vi "Ex3_Enums.vi"() -> ()   [LabVIEW 2024]
panel:
  in  "OK Button 2":bool
  out "Numeric 3":dbl
  in  "Numeric 2":dbl
  in  "Numeric":dbl
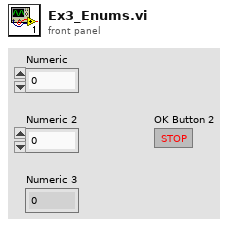
[diagram p1: front panel]
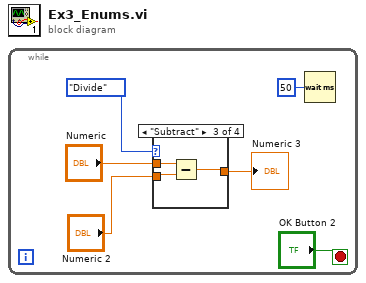
[diagram p0: block diagram]
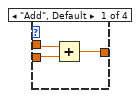
[diagram p2: hidden frame]
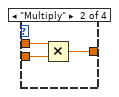
[diagram p3: hidden frame]
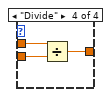
[diagram p4: hidden frame]
diagram:
  n1 = while {
    stop <- "OK Button 2" stop-if-true
    n2 = case shown="\"Subtract\"" enum16{"Add", "Subtract", "Multiply", "Divide"}."Divide" {
      tunnel: "Numeric 2" -> [w7 w12 w14 w17]
      tunnel: "Numeric" -> [w8 w11 w15 w16]
      tunnel: [w9 w10 w13 w18] -> w4
      frame "Add", Default {
        n3 = Add(x=w8, y=w7) -> (x+y=w9:dbl)
      }
      frame "Multiply" {
        n4 = Multiply(x=w11, y=w12) -> (x*y=w10:dbl)
      }
      frame "Subtract" {
        n5 = Subtract(x=w15, y=w14) -> (x-y=w13:dbl)
      }
      frame "Divide" {
        n6 = Divide(x=w16, y=w17) -> (x/y=w18:dbl)
      }
    }
    "Numeric 3" <- w4
    n7 = Wait (ms)(milliseconds to wait=u32 50) -> ()  [unwired: 1 out]
  }
